vi "add channel to SHM configuration.vi"(8 "error in":errorcluster, 10 "channel":refnum<class "TBM channel.lvclass">, 11 "SHM configuration in":refnum<class "Shared Memory configuration.lvclass">) -> (0 "error out":errorcluster, 3 "SHM configuration out":refnum<class "Shared Memory configuration.lvclass">)   [LabVIEW 2013, in "Shared Memory configuration.lvclass"]
uses:
  module/configuration/Shared Memory configuration.lvclass
  <vilib>/NI/Tag Bus Module Framework/channel/TBM channel.lvclass
  module/configuration/Shared Memory configuration.lvclass/Shared Memory configuration.ctl
  <vilib>/NI/Tag Bus/tag/tag descriptor.lvclass/tag descriptor.ctl
  <vilib>/NI/Tag Bus/tag/tag descriptor.lvclass
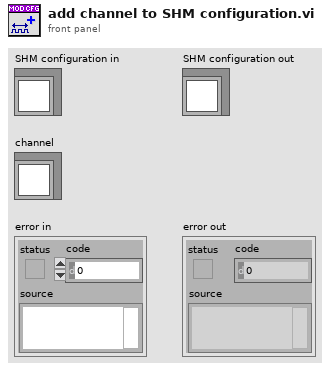
[diagram p1: front panel]
types:
  T1 = typedef "Shared Memory configuration.lvclass/Line.ctl" = cluster{"channel":refnum<class "TBM channel.lvclass">}
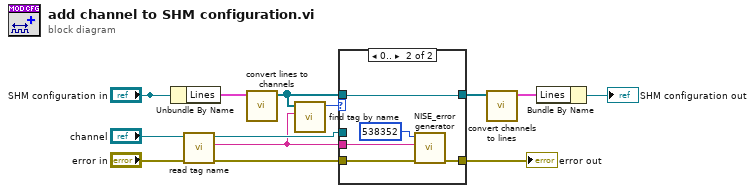
[diagram p0: block diagram]
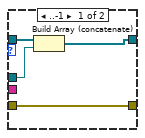
[diagram p2: hidden frame]
diagram:
  n1 = Unbundle By Name("SHM configuration in") -> ("Lines"=w6:T1[])
  n2 = call <vilib>:"read tag name.vi"("error in"="error in", "system tag in"="channel") -> ("error out"=w9:errorcluster, "name"=w4:string, "system tag out"=w7:refnum<class "TBM channel.lvclass">)  [unwired: 7 in]
  n3 = call "convert lines to channels.vi"("Lines in"=w6) -> ("channels out"=w5:refnum<class "TBM channel.lvclass">[])  [unwired: 9 in, 1 out]
  n4 = call <vilib>:"find tag by name.vi"("name"=w4, "tags in"=w5) -> ("index"=w10:i32)  [unwired: 9 in]
  n5 = case shown="0.." w10 {
    tunnel: w9 -> [w14 w21]
    tunnel: [w14 w20] -> w8
    tunnel: w4 -> [_ w19]
    tunnel: w5 -> [w17 w18]
    tunnel: w7 -> [w16 _]
    tunnel: [w15 w18] -> w3
    frame ..-1 {
      n6 = Build Array (concatenate)(w17, w16) -> (w15:refnum<class "TBM channel.lvclass">[])
    }
    frame 0.. {
      n7 = call <vilib>:"NISE_error generator.vi"("error in"=w21, "append error message"=w19, "error code (0)"=538352) -> ("error out"=w20:errorcluster)  [unwired: 6 in]
    }
  }
  "error out" <- w8
  n8 = call "convert channels to lines.vi"("channels"=w3) -> ("Lines"=w2:T1[])  [unwired: 9 in, 1 out]
  n9 = Bundle By Name(cluster="SHM configuration in", "Lines"=w2) -> (→"SHM configuration out":refnum<class "Shared Memory configuration.lvclass">)
